vi "update header UI.vi"(8 "error in (no error)":errorcluster, 9 "header ui refs":T1, 10 "engine in":refnum<class "Engine Parent Editor Node.lvclass">, 11 "shared memory editor node in":refnum<class "module editor node.lvclass">) -> (0 "error out":errorcluster, 2 "engine out":refnum<class "Engine Parent Editor Node.lvclass">, 3 "shared memory editor node out":refnum<class "module editor node.lvclass">)   [LabVIEW 2013, in "Shared Memory editor node.lvclass"]
uses:
  Shared Memory editor node.lvclass
  <vilib>/NI/DCAF/Tag Editor Core/Configuration Editor/Classes/Module editor node/module editor node.lvclass
  ui controls header.ctl
  <vilib>/NI/DCAF/Tag Editor Core/Configuration Editor/Classes/Engine Parent/Engine Parent Editor Node.lvclass
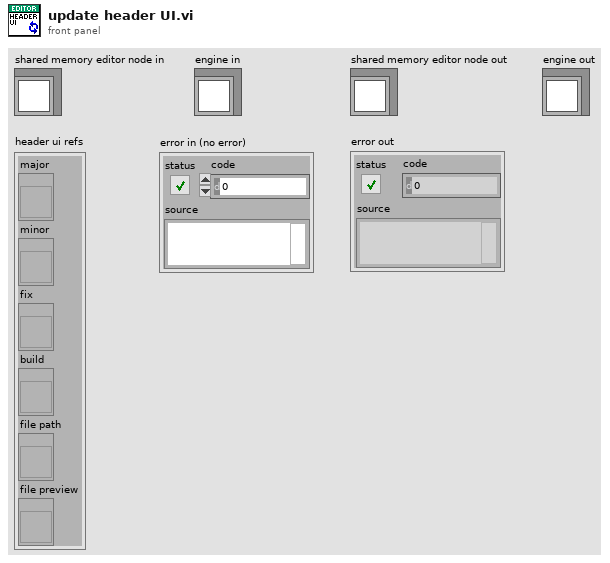
[diagram p1: front panel]
types:
  T1 = typedef "Shared Memory editor node.lvclass/ui controls header.ctl" = cluster{"major":refnum<vi>, "minor":refnum<vi>, "fix":refnum<vi>, "build":refnum<vi>, "file path":refnum<vi>, "file preview":refnum<vi>}
  T2 = cluster{"major":u16, "minor":u16, "fix":u16, "build":u16}
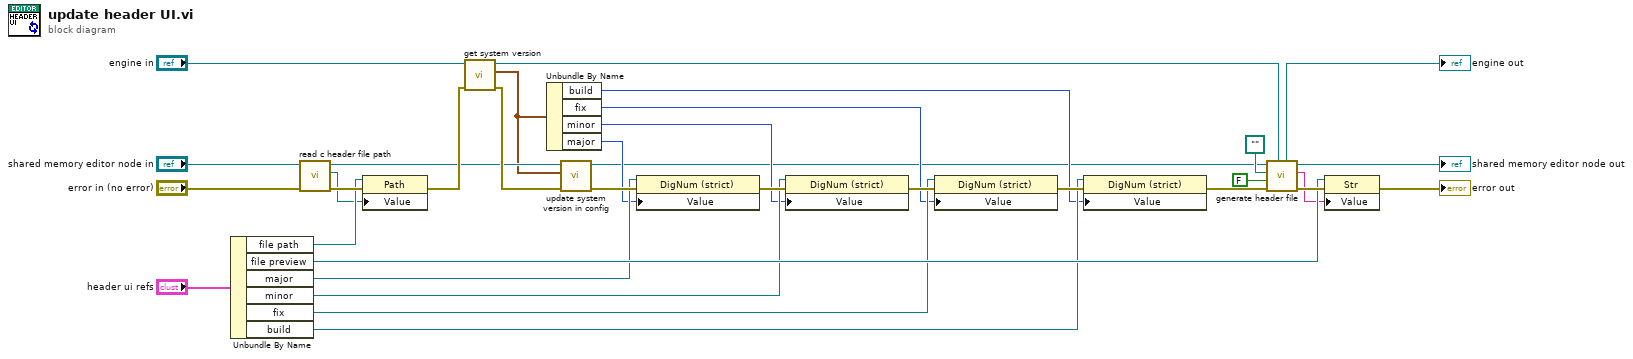
[diagram p0: block diagram]
diagram:
  n1 = Unbundle By Name("header ui refs") -> ("file path"=w30:refnum<vi>, "file preview"=w26:refnum<vi>, "major"=w9:refnum<vi>, "minor"=w6:refnum<vi>, "fix"=w8:refnum<vi>, "build"=w7:refnum<vi>)
  n2 = call "read c header file path.vi"("error in"="error in (no error)", "shared memory editor node"="shared memory editor node in") -> ("error out"=w31:errorcluster, "c header file path"=w25:path, "shared memory editor node out"=w16:refnum<class "module editor node.lvclass">)  [unwired: 7 in]
  n3 = property class="Path"(reference=w30, error in=w31, "Value"=w25) -> (error out=w21:errorcluster)  [unwired: 1 out]
  n4 = call "get system version.vi"("error in (no error)"=w21, "engine in"="engine in") -> ("error out"=w17:errorcluster, "version"=w15:T2, "engine out"=w19:refnum<class "Engine Parent Editor Node.lvclass">)  [unwired: 7 in]
  n5 = Unbundle By Name(w15) -> ("build"=w2:u16, "fix"=w3:u16, "minor"=w4:u16, "major"=w5:u16)
  n6 = call "update system version in config.vi"("error in"=w17, "version"=w15, "shared memory editor node"=w16) -> ("error out"=w14:errorcluster, "shared memory editor node out"=w1:refnum<class "module editor node.lvclass">)  [unwired: 7 in]
  n7 = property class="DigNum (strict)"(reference=w9, error in=w14, "Value"=w5) -> (error out=w13:errorcluster)  [unwired: 1 out]
  n8 = property class="DigNum (strict)"(reference=w6, error in=w13, "Value"=w4) -> (error out=w12:errorcluster)  [unwired: 1 out]
  n9 = property class="DigNum (strict)"(reference=w8, error in=w12, "Value"=w3) -> (error out=w11:errorcluster)  [unwired: 1 out]
  n10 = property class="DigNum (strict)"(reference=w7, error in=w11, "Value"=w2) -> (error out=w10:errorcluster)  [unwired: 1 out]
  n11 = call "generate header file.vi"("engine in"=w19, "error in (no error)"=w10, "write to file? (T)"=FALSE, "file path"=path "", "shared memory editor node in"=w1) -> ("error out"=w27:errorcluster, "generation output"=w24:string, "shared memory editor node out"=→"shared memory editor node out":refnum<class "module editor node.lvclass">, "engine out"=→"engine out":refnum<class "Engine Parent Editor Node.lvclass">)  [unwired: 3 in]
  n12 = property class="Str"(reference=w26, error in=w27, "Value"=w24) -> (error out=→"error out":errorcluster)  [unwired: 1 out]
